vi "Calculate Hold-In Measurements.vi"(0 "Stage Waveform Section":dbl[](array[numeric])) -> (4 "Max Stage":dbl, 6 "Min Stage":dbl, 8 "Avg Stage":dbl, 10 "Avg Max Stage":dbl, 15 "Avg Min Stage":dbl)   [LabVIEW 2019, in "Fuel Injector Analysis Addon Engine.lvlib"]
uses:
  Fuel Injector Analysis Addon Engine.lvlib
  <vilib>/Analysis/baseanly.llb/Mean (DBL).vi
  <vilib>/Analysis/NI_AALBase.lvlib
  <vilib>/Analysis/NI_AAL_SigProc.lvlib
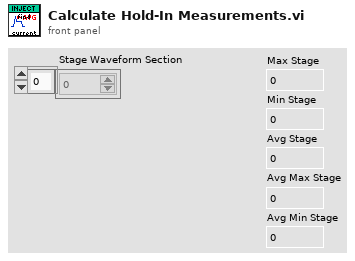
[diagram p1: front panel]
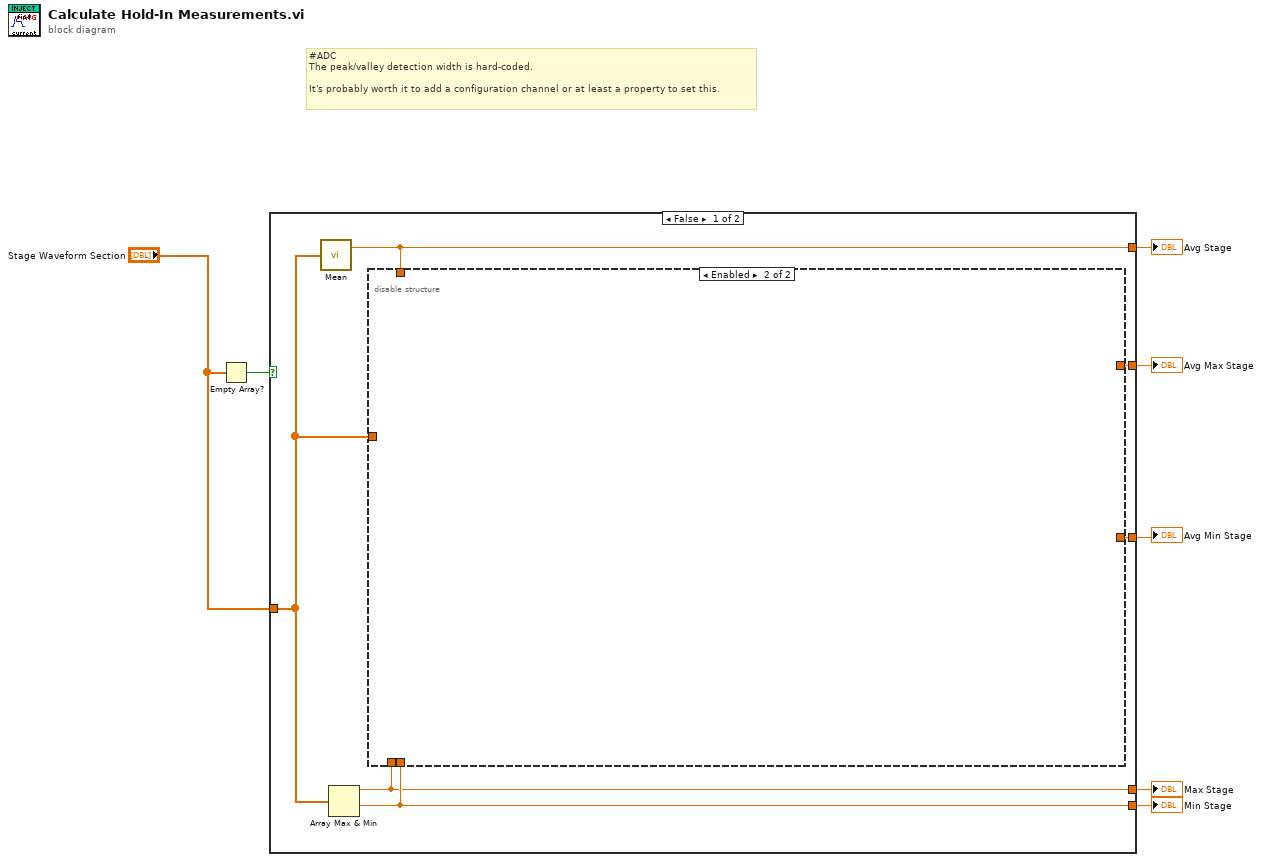
[diagram p0: block diagram]
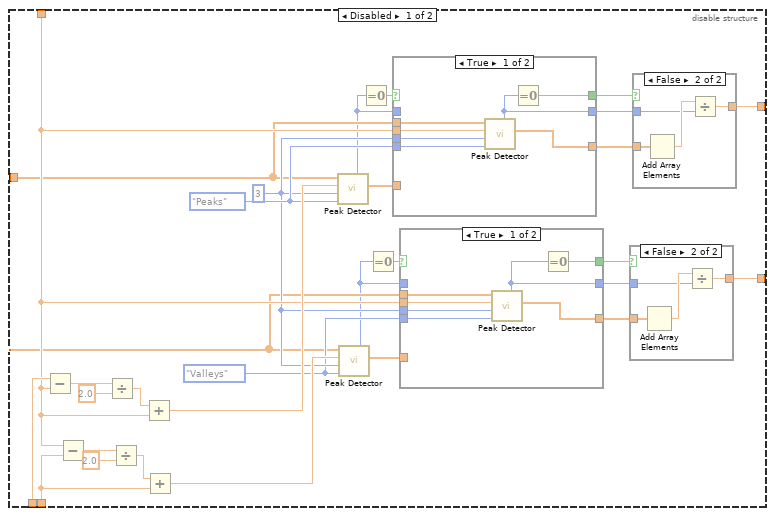
[diagram p2: hidden frame]
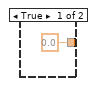
[diagram p3: hidden frame]
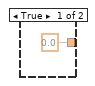
[diagram p4: hidden frame]
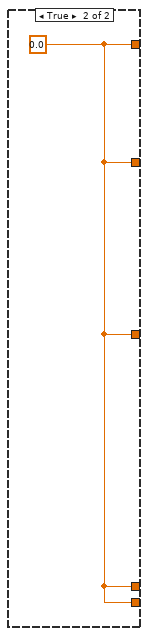
[diagram p7: hidden frame]
diagram:
  # "#ADC \nThe peak/valley detection width is hard-coded.\n\nIt's probably worth it to add a configuration channel or at least a property to set this."
  n1 = Empty Array?(array="Stage Waveform Section") -> (empty?=w1:bool)
  n2 = case shown="False" w1 {
    tunnel: [w13 w73] -> w7
    tunnel: [w8 w73] -> w6
    tunnel: [w12 w73] -> w5
    tunnel: [w11 w73] -> w4
    tunnel: [w10 w73] -> w3
    tunnel: "Stage Waveform Section" -> [w9 _]
    frame False {
      n3 = call-poly <vilib>:"Mean.vi"("X"=w9) -> ("mean"=w10:dbl)  [unwired: 1 out]
      n4 = Array Max & Min(array=w9) -> (max value=w11:dbl, min value=w12:dbl)  [unwired: 2 out]
      n5 = disable-structure shown="Enabled" {
        disable-tunnel: [w42 _] -> w13
        disable-tunnel: w12 -> [w39 _]
        disable-tunnel: w11 -> [w36 _]
        disable-tunnel: w10 -> [w27 _]
        disable-tunnel: w9 -> [w24 _]
        disable-tunnel: [w21 _] -> w8
        frame Disabled {
          w26 = 3 ("width")
          w25 = enum32{"Peaks", "Valleys"}."Valleys" ("peaks/valleys")
          w29 = enum32{"Peaks", "Valleys"}."Peaks" ("peaks/valleys")
          n6 = Subtract(x=w36, y=w27) -> (x-y=w33:dbl)
          n7 = Subtract(x=w27, y=w39) -> (x-y=w41:dbl)
          n8 = Divide(x=w33, y=2.0) -> (x/y=w35:dbl)
          n9 = Divide(x=w41, y=2.0) -> (x/y=w38:dbl)
          n10 = Add(x=w35, y=w27) -> (x+y=w32:dbl)
          n11 = Add(x=w38, y=w39) -> (x+y=w37:dbl)
          n12 = call <vilib>:"Peak Detector.vi"("peaks/valleys"=w29, "width"=w26, "threshold"=w32, "X"=w24) -> ("Amplitudes"=w30:dbl[], "# found"=w20:i32)  [unwired: 3 in, 3 out]
          n13 = call <vilib>:"Peak Detector.vi"("peaks/valleys"=w25, "width"=w26, "threshold"=w37, "X"=w24) -> ("Amplitudes"=w28:dbl[], "# found"=w17:i32)  [unwired: 3 in, 3 out]
          n14 = Equal To 0?(x=w20) -> (x = 0?=w19:bool)
          n15 = Equal To 0?(x=w17) -> (x = 0?=w16:bool)
          n16 = case shown="True" w19 {
            selector: w19 -> [_ w70]
            tunnel: w24 -> [w69 _]
            tunnel: [w68 w72] -> w31
            tunnel: w30 -> [_ w72]
            tunnel: [w64 w71] -> w23
            tunnel: w26 -> [w67 _]
            tunnel: w29 -> [w66 _]
            tunnel: w27 -> [w65 _]
            tunnel: w20 -> [_ w71]
            tunnel: [w63 w70] -> w18
            frame True {
              n17 = call <vilib>:"Peak Detector.vi"("peaks/valleys"=w66, "width"=w67, "threshold"=w65, "X"=w69) -> ("Amplitudes"=w68:dbl[], "# found"=w64:i32)  [unwired: 3 in, 3 out]
              n18 = Equal To 0?(x=w64) -> (x = 0?=w63:bool)
            }
            frame False {
            }
          }
          n19 = case shown="True" w16 {
            selector: w16 -> [_ w60]
            tunnel: w24 -> [w59 _]
            tunnel: [w58 w62] -> w22
            tunnel: w28 -> [_ w62]
            tunnel: [w54 w61] -> w15
            tunnel: w26 -> [w57 _]
            tunnel: w25 -> [w56 _]
            tunnel: w27 -> [w55 _]
            tunnel: w17 -> [_ w61]
            tunnel: [w53 w60] -> w14
            frame True {
              n20 = call <vilib>:"Peak Detector.vi"("peaks/valleys"=w56, "width"=w57, "threshold"=w55, "X"=w59) -> ("Amplitudes"=w58:dbl[], "# found"=w54:i32)  [unwired: 3 in, 3 out]
              n21 = Equal To 0?(x=w54) -> (x = 0?=w53:bool)
            }
            frame False {
            }
          }
          n22 = case shown="False" w14 {
            tunnel: [0.0 w47] -> w21
            tunnel: w22 -> [_ w45]
            tunnel: w15 -> [_ w44]
            frame True {
            }
            frame False {
              n23 = Add Array Elements(numeric array=w45) -> (sum=w46:dbl)
              n24 = Divide(x=w46, y=w44) -> (x/y=w47:dbl)
            }
          }
          n25 = case shown="False" w18 {
            tunnel: [0.0 w52] -> w42
            tunnel: w31 -> [_ w50]
            tunnel: w23 -> [_ w49]
            frame True {
            }
            frame False {
              n26 = Add Array Elements(numeric array=w50) -> (sum=w51:dbl)
              n27 = Divide(x=w51, y=w49) -> (x/y=w52:dbl)
            }
          }
        }
        frame Enabled {
        }
      }
    }
    frame True {
      w73 = 0.0 ("mean")
    }
  }
  "Avg Stage" <- w3
  "Avg Max Stage" <- w7
  "Max Stage" <- w4
  "Min Stage" <- w5
  "Avg Min Stage" <- w6
